vi "Parse Response Headers.vi"(11 "String":string) -> (3 "Response Headers":T1[](array[typedef]))   [LabVIEW 2015, in "NI_Azure_Blob.lvlib"]
uses:
  NI_Azure_Blob.lvlib
  Core/Name Value Pair.ctl
  Core/NI_Azure_Core.lvlib
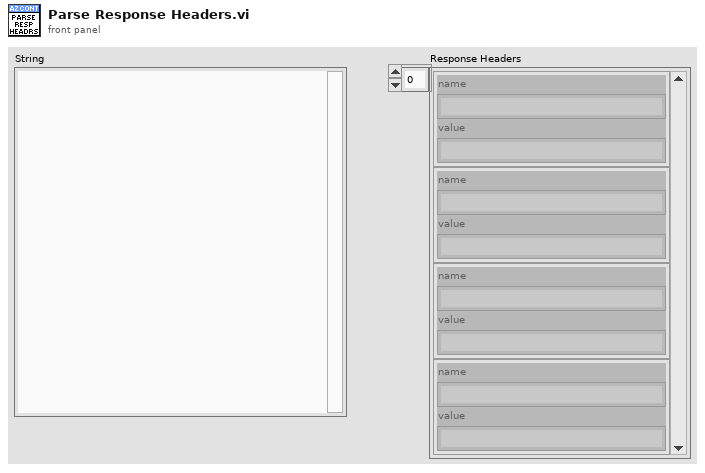
[diagram p1: front panel]
types:
  T1 = typedef "NI_Azure_Core.lvlib/Name Value Pair.ctl" = cluster{"name":string, "value":string}
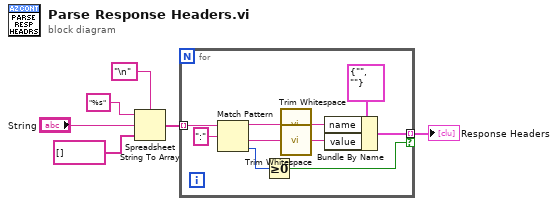
[diagram p0: block diagram]
diagram:
  n1 = Spreadsheet String To Array(delimiter (Tab)="\n", format string="%s", spreadsheet string="String", array type (2D Dbl)=string[] []) -> (array=w2:string[])
  n2 = for {
    tunnel: w2 -> [w16] mode=indexing
    tunnel: [w12] -> w1 mode=indexing if=w11
    n3 = Match Pattern(string=w16, regular expression=":") -> (before substring=w10:string, after substring=w9:string, offset past match=w14:i32)  [unwired: 1 in, 1 out]
    n4 = Greater Or Equal To 0?(x=w14) -> (x >= 0?=w11:bool)
    n5 = call <vilib>:"Trim Whitespace.vi"("string"=w10) -> ("trimmed string"=w7:string)  [unwired: 1 in]
    n6 = call <vilib>:"Trim Whitespace.vi"("string"=w9) -> ("trimmed string"=w8:string)  [unwired: 1 in]
    n7 = Bundle By Name(cluster=T1 {"name"="", "value"=""} ("Cluster"), "name"=w7, "value"=w8) -> (w12:T1)
  }
  "Response Headers" <- w1
